vi "Player Info.vi"(11 "Class":refnum<class "Shield Wall.lvclass">) -> (1 "Victory Speech":string, 2 "Name":string, 3 "Class":refnum<class "Shield Wall.lvclass">)   [LabVIEW 2015, in "Shield Wall.lvclass"]
uses:
  Shield Wall.lvclass
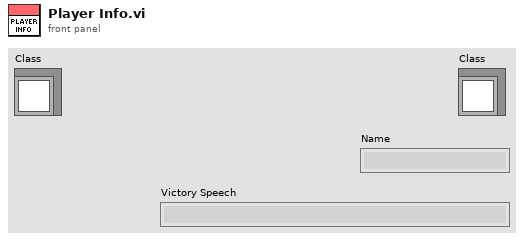
[diagram p1: front panel]
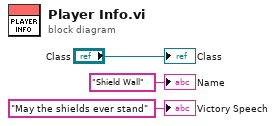
[diagram p0: block diagram]
diagram:
  "Class" <- "Class"
  "Name" <- "Shield Wall" ("Name")
  "Victory Speech" <- "May the shields ever stand" ("Victory Speech")
